vi "Rename All Class Controls.vi"(8 "Error In":errorcluster, 9 "new Name":string, 10 "old Name":string, 11 "Class Path":path) -> (0 "Error Out":errorcluster)   [LabVIEW 2011, in "Generator.lvlib"]
doc: "This VI renames all Class Controls which contains <B>old Name</B> with <B>new Name</B>."
uses:
  Generator.lvlib
  <vilib>/Utility/traverseref.llb/TRef TravTarget.ctl
  <vilib>/Utility/traverseref.llb/VI Scripting - Traverse.lvlib
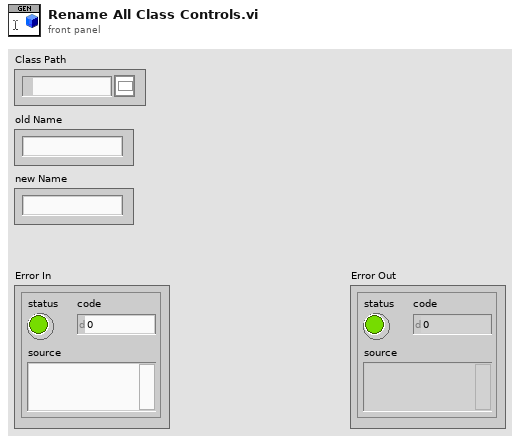
[diagram p1: front panel]
types:
  T1 = typedef "TRef TravTarget.ctl" = enum16{"FP", "BD", "Other"}
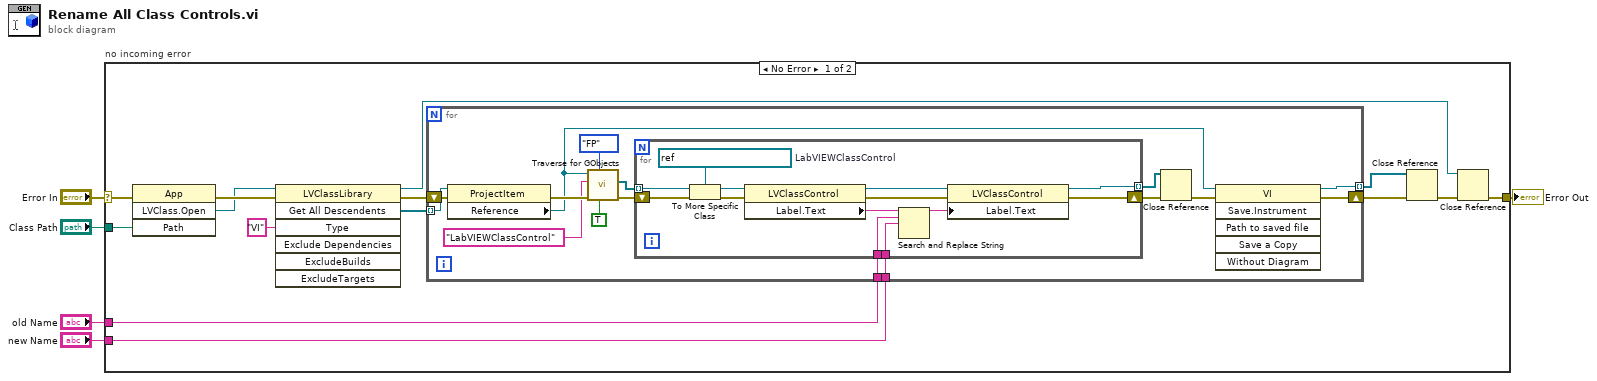
[diagram p0: block diagram]
diagram:
  n1 = case "no incoming error" shown="No Error" "Error In" {
    selector: "Error In" -> [w19 w48]
    tunnel: [w10 w48] -> w4
    tunnel: "Class Path" -> [w18 _]
    tunnel: "old Name" -> [w7 _]
    tunnel: "new Name" -> [w6 _]
    frame No Error {
      n2 = invoke class="App" method="LVClass.Open"(error in=w19, "Path"=w18) -> (error out=w17:errorcluster, "LVClass.Open"=w16:refnum<vi>)  [unwired: 2 in, 2 out]
      n3 = invoke class="LVClassLibrary" method="Get All Descendents"(reference=w16, error in=w17, "Type"="VI") -> (reference out=w9:refnum<vi>, error out=w14:errorcluster, "All Descendents"=w13:refnum<vi>[])  [unwired: 4 in, 4 out]
      n4 = for {
        tunnel: w13 -> [w34] mode=indexing
        shift-right: [w23] -> w12
        shift-left: w14 -> [w35]
        tunnel: [w24] -> w8 mode=indexing
        tunnel: w7 -> [w22]
        tunnel: w6 -> [w21]
        n5 = property class="ProjectItem"(reference=w34, error in=w35) -> (error out=w29:errorcluster, "Reference"=w26:refnum<vi>)  [unwired: 1 out]
        n6 = call <vilib>:"Traverse for GObjects.vi"("Traverse Generated Code (F)"=TRUE, "Traverse Target"=TRef_TravTarget."FP", "error in (no error)"=w29, "Class Name"="LabVIEWClassControl", "VI Refnum"=w26) -> ("error out"=w30:errorcluster, "References"=w31:refnum<vi>[])  [unwired: 3 in, 2 out]
        n7 = for {
          tunnel: w31 -> [w47] mode=indexing
          shift-right: [w39] -> w28
          shift-left: w30 -> [w44]
          tunnel: [w38] -> w27 mode=indexing
          tunnel: w22 -> [w37]
          tunnel: w21 -> [w36]
          w45 = refnum<vi> refnum  # LabVIEWClassControl
          n8 = To More Specific Class(target class=w45, reference=w47) -> (specific class reference=w46:refnum<vi>)  [unwired: 1 in, 1 out]
          n9 = property class="LVClassControl"(reference=w46, error in=w44) -> (reference out=w41:refnum<vi>, error out=w42:errorcluster, "Label.Text"=w43:string)
          n10 = Search and Replace String(input string=w43, search string=w37, replace string=w36) -> (result string=w40:string)  [unwired: 5 in, 3 out]
          n11 = property class="LVClassControl"(reference=w41, error in=w42, "Label.Text"=w40) -> (reference out=w38:refnum<vi>, error out=w39:errorcluster)
        }
        n12 = Close Reference(reference=w27, error in (no error)=w28) -> (error out=w25:errorcluster)
        n13 = invoke class="VI" method="Save.Instrument"(reference=w26, error in=w25) -> (reference out=w24:refnum<vi>, error out=w23:errorcluster)  [unwired: 4 in, 4 out]
      }
      n14 = Close Reference(reference=w8, error in (no error)=w12) -> (error out=w11:errorcluster)
      n15 = Close Reference(reference=w9, error in (no error)=w11) -> (error out=w10:errorcluster)
    }
    frame Error {
    }
  }
  "Error Out" <- w4
